vi "Get JSON CFG.vi"(11 "CFG JSON in":refnum<class "CFG JSON.lvclass">) -> (2 "<JSON> CFG":string, 3 "CFG JSON out":refnum<class "CFG JSON.lvclass">)   [LabVIEW 2024, in "HAL.lvlib" / "CFG JSON.lvclass"]
uses:
  CFG JSON.lvclass
  CFG JSON.lvclass/CFG JSON.ctl
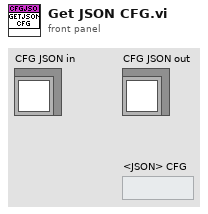
[diagram p1: front panel]
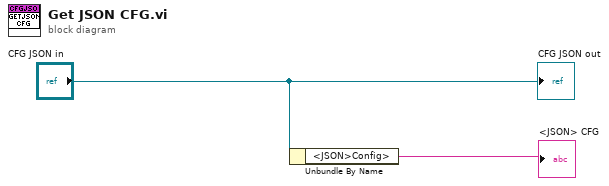
[diagram p0: block diagram]
diagram:
  n1 = Unbundle By Name("CFG JSON in") -> ("<JSON>Config>"=→"<JSON> CFG":string)
  "CFG JSON out" <- "CFG JSON in"
